vi "Percent VBus Scaling.vi"(9 "Min %VBus":dbl, 10 "Max %VBus":dbl, 11 "input (1 to -1)":dbl) -> (2 "output":dbl)   [LabVIEW 2014]
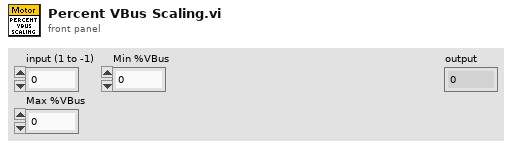
[diagram p1: front panel]
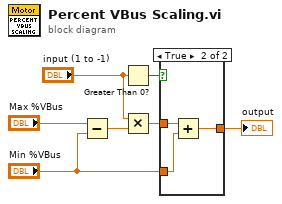
[diagram p0: block diagram]
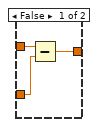
[diagram p2: hidden frame]
diagram:
  n1 = Subtract(x="Max %VBus", y="Min %VBus") -> (x-y=w6:dbl)
  n2 = Greater Than 0?(x="input (1 to -1)") -> (x > 0?=w7:bool)
  n3 = Multiply(x="input (1 to -1)", y=w6) -> (x*y=w5:dbl)
  n4 = case shown="True" w7 {
    tunnel: w5 -> [w10 w13]
    tunnel: [w8 w12] -> w4
    tunnel: "Min %VBus" -> [w9 w11]
    frame False {
      n5 = Subtract(x=w10, y=w9) -> (x-y=w8:dbl)
    }
    frame True {
      n6 = Add(x=w13, y=w11) -> (x+y=w12:dbl)
    }
  }
  "output" <- w4
